vi "Input_to_Array.vi"(8 "Numeric":i8, 11 "Array_In":i8[](array[numeric])) -> (3 "Array_Out":i8[](array[numeric]))   [LabVIEW 2020]
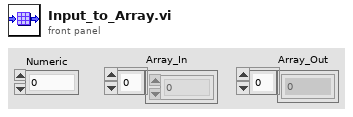
[diagram p1: front panel]
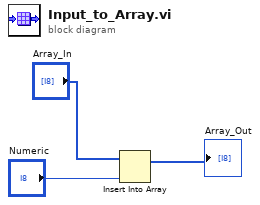
[diagram p0: block diagram]
diagram:
  n1 = Insert Into Array(array="Array_In", new element="Numeric") -> (→"Array_Out":i8[])  [unwired: 1 in]
